vi "Main FPGA.vi"() -> ()   [LabVIEW 2025]
uses:
  <vilib>/rvi/Emulation/niFpgaGetClockAttributes.vi
  <vilib>/rvi/Emulation/niFpgaSctlEmulationGetInTimedLoop.vi
  <vilib>/rvi/Emulation/niFpgaEmulationReportErrorSimple.vi
  <vilib>/rvi/eio/common/nirviEmuTemplateMethod_errors.vi
  <vilib>/rvi/Emulation/niFpgaCriticalErrorInLSC.vi
  <vilib>/eio/EIONode/EIONode.xnode
panel:
  in  "Count(mSec)":u32
  in  "LED3":bool
  in  "LED2":bool
  in  "LED1":bool
  in  "LED0":bool
  out "Button0":bool
  out "AccelerationX":i16
  out "AccelerationY":i16
  out "AccelerationZ":i16
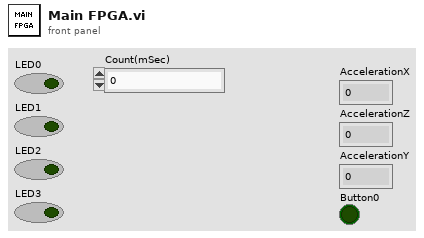
[diagram p1: front panel]
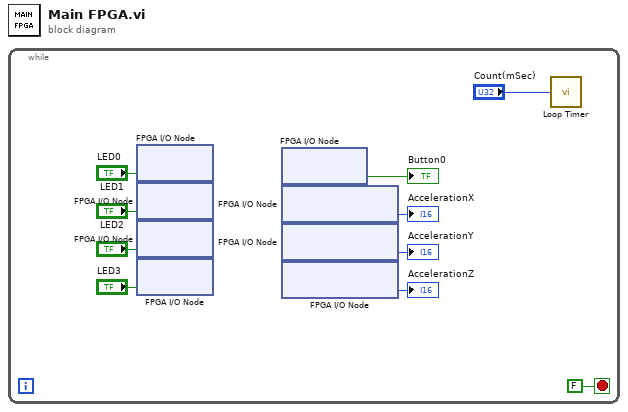
[diagram p0: block diagram]
diagram:
  n1 = while {
    stop <- FALSE stop-if-true
    n2 = xnode "FPGA I/O Node"("LED0"="LED0") -> ()  [unwired: 1 in, 1 out]
    n3 = xnode "FPGA I/O Node"("LED1"="LED1") -> ()  [unwired: 1 in, 1 out]
    n4 = xnode "FPGA I/O Node"("LED2"="LED2") -> ()  [unwired: 1 in, 1 out]
    n5 = xnode "FPGA I/O Node"("LED3"="LED3") -> ()  [unwired: 1 in, 1 out]
    n6 = xnode "FPGA I/O Node"() -> ("Button0"=→"Button0":bool)  [unwired: 1 in, 1 out]
    n7 = xnode "FPGA I/O Node"() -> ("AccelerationX"=→"AccelerationX":i16)  [unwired: 1 in, 1 out]
    n8 = xnode "FPGA I/O Node"() -> ("AccelerationY"=→"AccelerationY":i16)  [unwired: 1 in, 1 out]
    n9 = xnode "FPGA I/O Node"() -> ("AccelerationZ"=→"AccelerationZ":i16)  [unwired: 1 in, 1 out]
    n10 = call "Loop Timer"("Count(mSec)"="Count(mSec)") -> ()  [unwired: 1 out]
  }
